vi "AccurateTickCount.vi"() -> (0 "seconds":dbl)   [LabVIEW 2011]
uses:
  kernel32.dll
panel:
  out "freq":u64
  out "count":u64
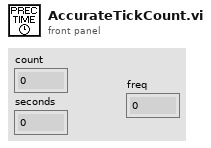
[diagram p1: front panel]
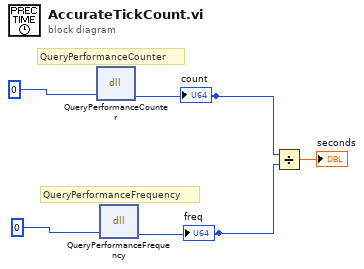
[diagram p0: block diagram]
diagram:
  # "QueryPerformanceFrequency"
  # "QueryPerformanceCounter"
  n1 = dll-call lib="kernel32.dll" fn="QueryPerformanceCounter"("frequency"=u64 0) -> ("frequency"=w2:u64)  [unwired: 4 in, 2 out]
  "count" <- w2
  n2 = dll-call lib="kernel32.dll" fn="QueryPerformanceFrequency"("frequency"=u64 0) -> ("frequency"=w3:u64)  [unwired: 4 in, 2 out]
  "freq" <- w3
  n3 = Divide(x=w2, y=w3) -> (x/y=→"seconds":dbl)
